vi "SV TDMS Read Octave Info.vi"(8 "error in":errorcluster, 9 "channel name in":string, 10 "group name in":string, 11 "tdms file":refnum<k34>) -> (0 "error out":errorcluster, 1 "channel name out":string, 2 "group name out":string, 3 "tdms file out":refnum<k34>, 4 "octave info":T2 {"engineering units" items=["custom..."=0, "V"=1, "A"=21, "C"=30, "pC"=31, "s"=32, "-"=29, "Pa"=2, "N"=20, "g"=3, "m/s^2"=4, "m/s"=5, "m"=6, "mm/s"=12, "mm"=13, "micron/s"=14, "micron"=15, "in/s^2"=7, "in/s"=8, "in"=9, "mil/s"=10, "mil"=11, "rad/s^2"=16, "rad/s"=17, "rad"=18, "deg/s^2"=26, "deg/s"=27, "deg"=28, "RPM"=22, "cycle/s^2"=23, "Hz"=24, "cycle"=25, "strain"=19]; "dB reference" format="%.2e"; "weighting filter" items=["Linear", "A-weighting", "B-weighting", "C-weighting", "ITU-R 468-4", "Dolby", "CCITT", "C-message", "Wb", "Wc", "Wd", "We", "Wf", "Wh", "Wj", "Wk", "Wm", "AES17 20 kHz lowpass", "AES17 40 kHz lowpass", "AES17 20 kHz highpass", "AES17 40 kHz highpass"]}, 6 "labels":T1)   [LabVIEW 2017]
uses:
  <vilib>/addons/_NISVFA/_Shared subVIs/Controls/svc_Octave Info.ctl
  <vilib>/addons/_NISVFA/_Shared subVIs/Controls/svc_Octave Standard.ctl
  <vilib>/addons/_NISVFA/_Shared subVIs/Controls/svc_Weighting Filter Text Ring.ctl
  <vilib>/addons/_NISVFA/_Shared subVIs/Controls/svc_Engineering Units Text Ring.ctl
  <vilib>/addons/_NISVFA/_Shared subVIs/Controls/NI Channel Properties.ctl
  <vilib>/addons/_NISVFA/_Shared subVIs/Controls/SV Channel Properties.ctl
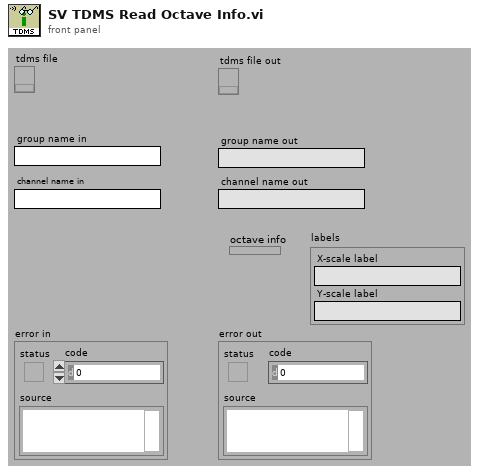
[diagram p1: front panel]
types:
  T1 = cluster{"X-scale label":string, "Y-scale label":string}
  T2 = typedef "svc_Octave Info.ctl" = cluster{"standard":T3, "bandwidth":enum16{"1 octave", "1/3 octave", "1/6 octave", "1/12 octave", "1/24 octave"}, "low band":i32, "high band":i32, "weighting filter":T4, "dB reference":dbl, "dB On":bool, "unit label":string, "channel name":string, "description":string, "engineering units":T5, "custom label":string, "spectrum type":enum16{"power", "magnitude"}, "spectral density":bool, "filters settled":bool}
  T3 = typedef "svc_Octave Standard.ctl" = enum16{"ANSI S1.11", "IEC 61260"}
  T4 = typedef "svc_Weighting Filter Text Ring.ctl" = u16
  T5 = typedef "svc_Engineering Units Text Ring.ctl" = u16
  T6 = typedef "NI Channel Properties.ctl" = u16
  T7 = typedef "SV Channel Properties.ctl" = u16
  T8 = enum16{"1 octave", "1/3 octave", "1/6 octave", "1/12 octave", "1/24 octave"}
  T9 = cluster{"scale label with units":string, "scale label with units":string}
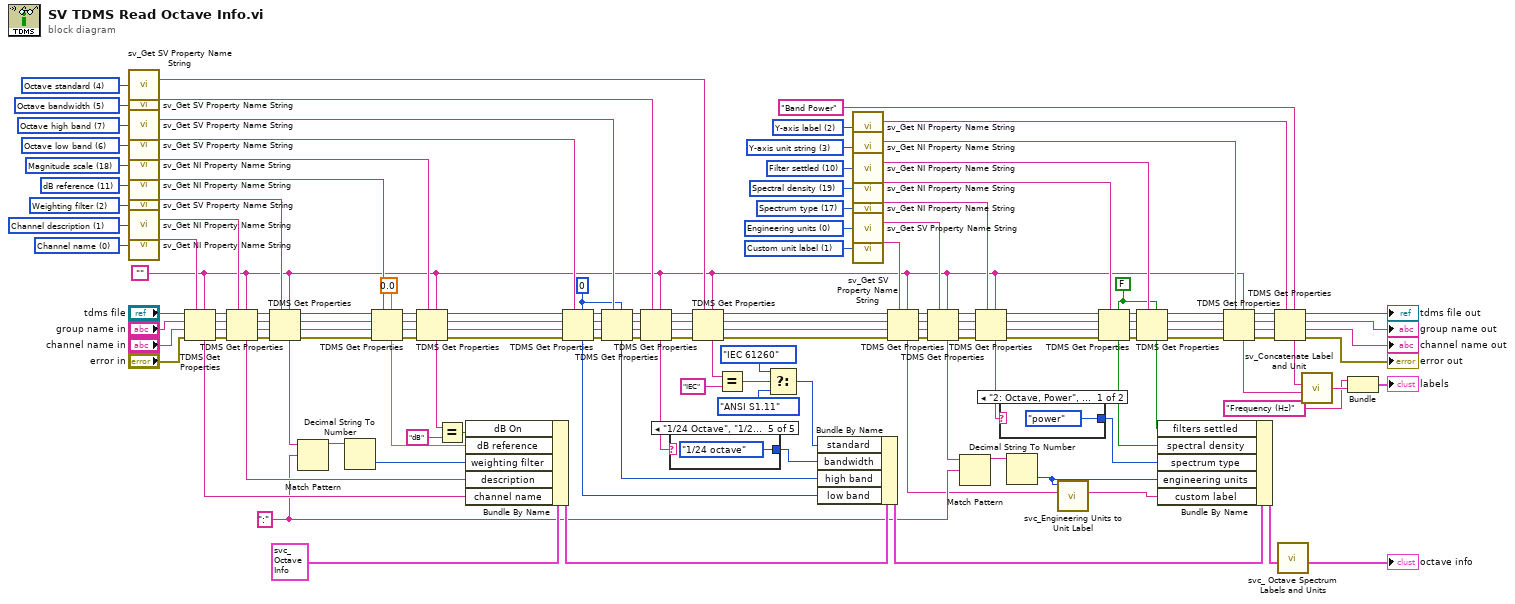
[diagram p0: block diagram]
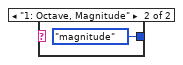
[diagram p2: hidden frame]
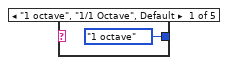
[diagram p3: hidden frame]
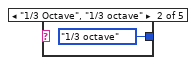
[diagram p4: hidden frame]
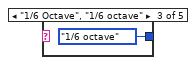
[diagram p5: hidden frame]
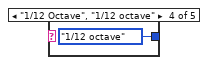
[diagram p6: hidden frame]
diagram:
  w7 = FALSE ("spectral density")
  w29 = 0 ("high band")
  w11 = ":" ("regular expression")
  w10 = ""
  w64 = T6 17 items=["Channel name", "Channel description", "Y-axis label", "Y-axis unit string", "X-axis label", "X-axis unit string", "x0", "dx", "Number of samples", "X channel", "Filter settled", "dB reference", "Window", "Window parameter", "Window size", "FFT size", "Peak units", "Spectrum type", "Magnitude scale", "Spectral density"] ("property")
  w86 = T7 1 items=["Engineering units", "Custom unit label", "Weighting filter", "Pregain", "Octave standard", "Octave bandwidth", "Octave low band", "Octave high band", "Spectrum skewed"] ("SV property")
  w73 = T7 4 items=["Engineering units", "Custom unit label", "Weighting filter", "Pregain", "Octave standard", "Octave bandwidth", "Octave low band", "Octave high band", "Spectrum skewed"] ("SV property")
  w74 = T7 5 items=["Engineering units", "Custom unit label", "Weighting filter", "Pregain", "Octave standard", "Octave bandwidth", "Octave low band", "Octave high band", "Spectrum skewed"] ("SV property")
  w84 = T7 7 items=["Engineering units", "Custom unit label", "Weighting filter", "Pregain", "Octave standard", "Octave bandwidth", "Octave low band", "Octave high band", "Spectrum skewed"] ("SV property")
  w85 = T7 6 items=["Engineering units", "Custom unit label", "Weighting filter", "Pregain", "Octave standard", "Octave bandwidth", "Octave low band", "Octave high band", "Spectrum skewed"] ("SV property")
  w88 = T7 0 items=["Engineering units", "Custom unit label", "Weighting filter", "Pregain", "Octave standard", "Octave bandwidth", "Octave low band", "Octave high band", "Spectrum skewed"] ("SV property")
  w75 = T7 2 items=["Engineering units", "Custom unit label", "Weighting filter", "Pregain", "Octave standard", "Octave bandwidth", "Octave low band", "Octave high band", "Spectrum skewed"] ("SV property")
  w78 = T6 11 items=["Channel name", "Channel description", "Y-axis label", "Y-axis unit string", "X-axis label", "X-axis unit string", "x0", "dx", "Number of samples", "X channel", "Filter settled", "dB reference", "Window", "Window parameter", "Window size", "FFT size", "Peak units", "Spectrum type", "Magnitude scale", "Spectral density"] ("property")
  w79 = T6 2 items=["Channel name", "Channel description", "Y-axis label", "Y-axis unit string", "X-axis label", "X-axis unit string", "x0", "dx", "Number of samples", "X channel", "Filter settled", "dB reference", "Window", "Window parameter", "Window size", "FFT size", "Peak units", "Spectrum type", "Magnitude scale", "Spectral density"] ("property")
  w80 = T6 3 items=["Channel name", "Channel description", "Y-axis label", "Y-axis unit string", "X-axis label", "X-axis unit string", "x0", "dx", "Number of samples", "X channel", "Filter settled", "dB reference", "Window", "Window parameter", "Window size", "FFT size", "Peak units", "Spectrum type", "Magnitude scale", "Spectral density"] ("property")
  w82 = T6 0 items=["Channel name", "Channel description", "Y-axis label", "Y-axis unit string", "X-axis label", "X-axis unit string", "x0", "dx", "Number of samples", "X channel", "Filter settled", "dB reference", "Window", "Window parameter", "Window size", "FFT size", "Peak units", "Spectrum type", "Magnitude scale", "Spectral density"] ("property")
  w81 = T6 1 items=["Channel name", "Channel description", "Y-axis label", "Y-axis unit string", "X-axis label", "X-axis unit string", "x0", "dx", "Number of samples", "X channel", "Filter settled", "dB reference", "Window", "Window parameter", "Window size", "FFT size", "Peak units", "Spectrum type", "Magnitude scale", "Spectral density"] ("property")
  w83 = T6 18 items=["Channel name", "Channel description", "Y-axis label", "Y-axis unit string", "X-axis label", "X-axis unit string", "x0", "dx", "Number of samples", "X channel", "Filter settled", "dB reference", "Window", "Window parameter", "Window size", "FFT size", "Peak units", "Spectrum type", "Magnitude scale", "Spectral density"] ("property")
  w87 = T6 19 items=["Channel name", "Channel description", "Y-axis label", "Y-axis unit string", "X-axis label", "X-axis unit string", "x0", "dx", "Number of samples", "X channel", "Filter settled", "dB reference", "Window", "Window parameter", "Window size", "FFT size", "Peak units", "Spectrum type", "Magnitude scale", "Spectral density"] ("property")
  w89 = T6 10 items=["Channel name", "Channel description", "Y-axis label", "Y-axis unit string", "X-axis label", "X-axis unit string", "x0", "dx", "Number of samples", "X channel", "Filter settled", "dB reference", "Window", "Window parameter", "Window size", "FFT size", "Peak units", "Spectrum type", "Magnitude scale", "Spectral density"] ("property")
  n1 = call <vilib>:"sv_Get SV Property Name String.vi"("property"=w73) -> ("TDMS property name"=w67:string)  [unwired: 13 in, 1 out]
  n2 = call <vilib>:"sv_Get SV Property Name String.vi"("property"=w74) -> ("TDMS property name"=w68:string)  [unwired: 13 in, 1 out]
  n3 = call <vilib>:"sv_Get SV Property Name String.vi"("property"=w84) -> ("TDMS property name"=w30:string)  [unwired: 13 in, 1 out]
  n4 = call <vilib>:"sv_Get SV Property Name String.vi"("property"=w85) -> ("TDMS property name"=w31:string)  [unwired: 13 in, 1 out]
  n5 = call <vilib>:"sv_Get NI Property Name String.vi"("property"=w83) -> ("TDMS property name"=w35:string)  [unwired: 13 in, 1 out]
  n6 = call <vilib>:"sv_Get NI Property Name String.vi"("property"=w78) -> ("TDMS property name"=w69:string)  [unwired: 13 in, 1 out]
  n7 = call <vilib>:"sv_Get SV Property Name String.vi"("property"=w75) -> ("TDMS property name"=w70:string)  [unwired: 13 in, 1 out]
  n8 = call <vilib>:"sv_Get NI Property Name String.vi"("property"=w81) -> ("TDMS property name"=w71:string)  [unwired: 13 in, 1 out]
  n9 = call <vilib>:"sv_Get NI Property Name String.vi"("property"=w82) -> ("TDMS property name"=w72:string)  [unwired: 13 in, 1 out]
  n10 = TDMS Get Properties(5:w10, 7:w72, 8:"error in", 9:"channel name in", 10:"group name in", 11:"tdms file") -> (0:w118:errorcluster, 1:w121:string, 2:w120:string, 3:w119:refnum<k34>, 4:w60:string)  [unwired: 1 out]
  n11 = TDMS Get Properties(5:w10, 7:w71, 8:w118, 9:w121, 10:w120, 11:w119) -> (0:w56:errorcluster, 1:w55:string, 2:w54:string, 3:w53:refnum<k34>, 4:w59:string)  [unwired: 1 out]
  n12 = TDMS Get Properties(5:w10, 7:w70, 8:w56, 9:w55, 10:w54, 11:w53) -> (0:w90:errorcluster, 1:w91:string, 2:w92:string, 3:w93:refnum<k34>, 4:w39:string)  [unwired: 1 out]
  n13 = Match Pattern(string=w39, regular expression=w11) -> (before substring=w40:string)  [unwired: 1 in, 3 out]
  n14 = Decimal String To Number(string=w40) -> (number=w38:i32)  [unwired: 2 in, 1 out]
  n15 = TDMS Get Properties(5:0.0 ("dB reference"), 7:w69, 8:w90, 9:w91, 10:w92, 11:w93) -> (0:w110:errorcluster, 1:w111:string, 2:w112:string, 3:w113:refnum<k34>, 4:w36:dbl)  [unwired: 1 out]
  n16 = TDMS Get Properties(5:w10, 7:w35, 8:w110, 9:w111, 10:w112, 11:w113) -> (0:w133:errorcluster, 1:w132:string, 2:w131:string, 3:w130:refnum<k34>, 4:w33:string)  [unwired: 1 out]
  n17 = Equal?(x=w33, y="dB" ("regular expression")) -> (x = y?=w32:bool)
  n18 = Bundle By Name(cluster=T2 {"standard"=enum."ANSI S1.11", "bandwidth"=enum."1 octave", "low band"=0, "high band"=0, "weighting filter"=0, "dB reference"=0.0, "dB On"=FALSE, "unit label"="", "channel name"="", "description"="", "engineering units"=0, "custom label"="", "spectrum type"=enum."power", "spectral density"=FALSE, "filters settled"=FALSE} ("octave info"), "dB On"=w32, "dB reference"=w36, "weighting filter"=w38, "description"=w59, "channel name"=w60) -> (w26:T2)
  n19 = TDMS Get Properties(5:w29, 7:w31, 8:w133, 9:w132, 10:w131, 11:w130) -> (0:w126:errorcluster, 1:w129:string, 2:w128:string, 3:w127:refnum<k34>, 4:w28:i32)  [unwired: 1 out]
  n20 = TDMS Get Properties(5:w29, 7:w30, 8:w126, 9:w129, 10:w128, 11:w127) -> (0:w125:errorcluster, 1:w124:string, 2:w123:string, 3:w122:refnum<k34>, 4:w27:i32)  [unwired: 1 out]
  n21 = TDMS Get Properties(5:w10, 7:w68, 8:w125, 9:w124, 10:w123, 11:w122) -> (0:w117:errorcluster, 1:w116:string, 2:w115:string, 3:w114:refnum<k34>, 4:w25:string)  [unwired: 1 out]
  n22 = case shown="\"1/24 Octave\", \"1/24 octave\"" w25 {
    tunnel: [T8."1 octave" ("bandwidth") T8."1/3 octave" ("bandwidth") T8."1/6 octave" ("bandwidth") T8."1/12 octave" ("bandwidth") T8."1/24 octave" ("bandwidth")] -> w24
    frame "1 octave", "1/1 Octave", Default {
    }
    frame "1/3 Octave", "1/3 octave" {
    }
    frame "1/6 Octave", "1/6 octave" {
    }
    frame "1/12 Octave", "1/12 octave" {
    }
    frame "1/24 Octave", "1/24 octave" {
    }
  }
  n23 = TDMS Get Properties(5:w10, 7:w67, 8:w117, 9:w116, 10:w115, 11:w114) -> (0:w102:errorcluster, 1:w103:string, 2:w104:string, 3:w105:refnum<k34>, 4:w23:string)  [unwired: 1 out]
  n24 = Equal?(x=w23, y="IEC") -> (x = y?=w21:bool)
  n25 = Select(t=svc_Octave_Standard."IEC 61260" ("standard"), s=w21, f=svc_Octave_Standard."ANSI S1.11" ("standard")) -> (s? t:f=w18:T3)
  n26 = Bundle By Name(cluster=w26, "standard"=w18, "bandwidth"=w24, "high band"=w27, "low band"=w28) -> (w15:T2)
  n27 = call <vilib>:"sv_Get NI Property Name String.vi"("property"=w79) -> ("TDMS property name"=w58:string)  [unwired: 13 in, 1 out]
  n28 = call <vilib>:"sv_Get NI Property Name String.vi"("property"=w80) -> ("TDMS property name"=w44:string)  [unwired: 13 in, 1 out]
  n29 = call <vilib>:"sv_Get NI Property Name String.vi"("property"=w89) -> ("TDMS property name"=w77:string)  [unwired: 13 in, 1 out]
  n30 = call <vilib>:"sv_Get NI Property Name String.vi"("property"=w87) -> ("TDMS property name"=w76:string)  [unwired: 13 in, 1 out]
  n31 = call <vilib>:"sv_Get NI Property Name String.vi"("property"=w64) -> ("TDMS property name"=w63:string)  [unwired: 13 in, 1 out]
  n32 = call <vilib>:"sv_Get SV Property Name String.vi"("property"=w88) -> ("TDMS property name"=w65:string)  [unwired: 13 in, 1 out]
  n33 = call <vilib>:"sv_Get SV Property Name String.vi"("property"=w86) -> ("TDMS property name"=w66:string)  [unwired: 13 in, 1 out]
  n34 = TDMS Get Properties(5:w10, 7:w66, 8:w102, 9:w103, 10:w104, 11:w105) -> (0:w98:errorcluster, 1:w99:string, 2:w100:string, 3:w101:refnum<k34>, 4:w4:string)  [unwired: 1 out]
  n35 = TDMS Get Properties(5:w10, 7:w65, 8:w98, 9:w99, 10:w100, 11:w101) -> (0:w94:errorcluster, 1:w95:string, 2:w96:string, 3:w97:refnum<k34>, 4:w12:string)  [unwired: 1 out]
  n36 = Match Pattern(string=w12, regular expression=w11) -> (before substring=w13:string)  [unwired: 1 in, 3 out]
  n37 = TDMS Get Properties(5:w10, 7:w63, 8:w94, 9:w95, 10:w96, 11:w97) -> (0:w137:errorcluster, 1:w136:string, 2:w135:string, 3:w134:refnum<k34>, 4:w9:string)  [unwired: 1 out]
  n38 = case shown="\"2: Octave, Power\", Default" w9 {
    tunnel: [enum16{"power", "magnitude"}."power" ("spectrum type") enum16{"power", "magnitude"}."magnitude" ("spectrum type")] -> w8
    frame "2: Octave, Power", Default {
    }
    frame "1: Octave, Magnitude" {
    }
  }
  n39 = Decimal String To Number(string=w13) -> (number=w2:i32)  [unwired: 2 in, 1 out]
  n40 = call <vilib>:"svc_Engineering Units to Unit Label.vi"("custom label"=w4, "engineering units"=w2) -> ("unit label"=w3:string)  [unwired: 8 in, 1 out]
  n41 = TDMS Get Properties(5:w7, 7:w76, 8:w137, 9:w136, 10:w135, 11:w134) -> (0:w138:errorcluster, 1:w139:string, 2:w140:string, 3:w141:refnum<k34>, 4:w5:bool)  [unwired: 1 out]
  n42 = TDMS Get Properties(5:w7, 7:w77, 8:w138, 9:w139, 10:w140, 11:w141) -> (0:w52:errorcluster, 1:w51:string, 2:w50:string, 3:w49:refnum<k34>, 4:w6:bool)  [unwired: 1 out]
  n43 = Bundle By Name(cluster=w15, "filters settled"=w6, "spectral density"=w5, "spectrum type"=w8, "engineering units"=w2, "custom label"=w3) -> (w14:T2)
  n44 = TDMS Get Properties(5:w10, 7:w44, 8:w52, 9:w51, 10:w50, 11:w49) -> (0:w45:errorcluster, 1:w46:string, 2:w47:string, 3:w48:refnum<k34>, 4:w42:string)  [unwired: 1 out]
  "group name out" <- w47
  "channel name out" <- w46
  "tdms file out" <- w48
  n45 = TDMS Get Properties(5:"Band Power" ("channel name"), 7:w58, 8:w45, 9:w46, 10:w47, 11:w48) -> (0:→"error out":errorcluster, 4:w43:string)  [unwired: 4 out]
  n46 = call <vilib>:"svc_ Octave Spectrum Labels and Units.vi"("octave info"=w14) -> ("octave info out"=→"octave info":T2)  [unwired: 9 in, 1 out]
  n47 = call <vilib>:"sv_Concatenate Label and Unit.vi"("unit string"=w42, "label"=w43) -> ("scale label with units"=w41:string)  [unwired: 4 in]
  n48 = Bundle("scale label with units"="Frequency (Hz)", "scale label with units"=w41) -> (→"labels":T9)  [unwired: 1 in]
